vi "VsEp-Plot Metrics.vi"(3 "error in (no error)":errorcluster, 4 "metrics":dbl[][](array[numeric]), 5 "level":dbl[](array[numeric])) -> (0 "error out":errorcluster, 1 "appended array":cluster{"array":ext[], "array":ext[]}[](array[cluster]))   [LabVIEW 2020]
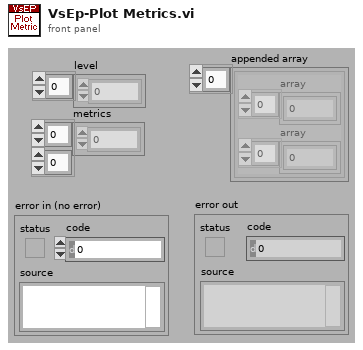
[diagram p1: front panel]
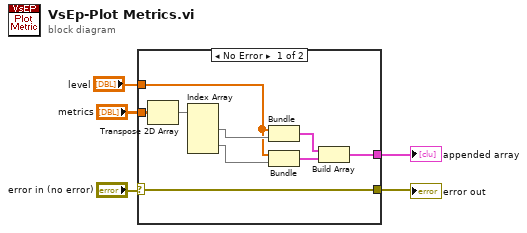
[diagram p0: block diagram]
diagram:
  n1 = case shown="No Error" "error in (no error)" {
    selector: "error in (no error)" -> [w10 w15]
    tunnel: "metrics" -> [w12 _]
    tunnel: [w11 _] -> w4
    tunnel: [w10 w15] -> w2
    tunnel: "level" -> [w6 _]
    frame No Error {
      n2 = Transpose 2D Array(2D array=w12) -> (transposed array=w9:dbl[][])
      n3 = Index Array(array=w9) -> (element #1=w8:dbl[], element #2=w7:dbl[])  [unwired: 4 in]
      n4 = Bundle("level"=w6, w8) -> (w14:cluster{"level":dbl[], dbl[]})  [unwired: 1 in]
      n5 = Bundle("level"=w6, w7) -> (w13:cluster{"level":dbl[], dbl[]})  [unwired: 1 in]
      n6 = Build Array(w14, w13) -> (w11:cluster{"level":dbl[], dbl[]}[])
    }
    frame Error {
    }
  }
  "appended array" <- w4
  "error out" <- w2
